vi "measure_voltage_lasers.vi"(8 "rate":dbl=100.0, 10 "number of samples":i32=100) -> (1 "data":dynamicdata(graph), 2 "Detected Voltage":string, 3 "Incident Voltage":string)   [LabVIEW 2017]
uses:
  <vilib>/Analysis/baseanly.llb/Mean (DBL).vi
  <vilib>/Analysis/NI_AALBase.lvlib
panel:
  out "Waveform Graph 2":dynamicdata(graph)
  out "Waveform Graph":dynamicdata(graph)
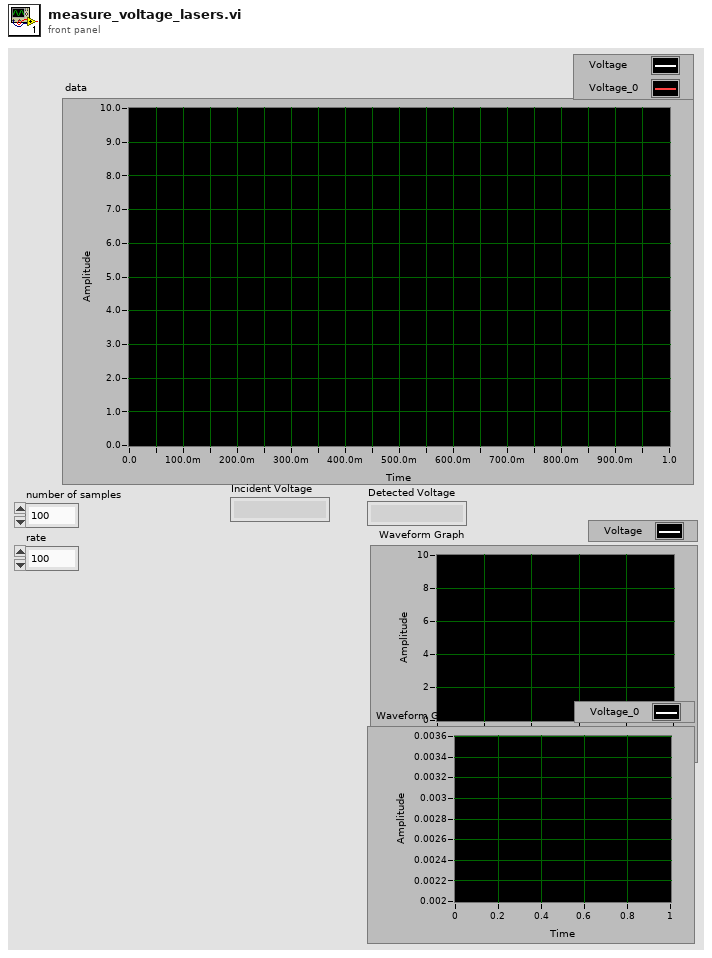
[diagram p1: front panel]
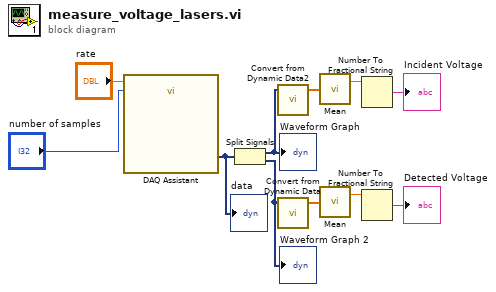
[diagram p0: block diagram]
diagram:
  n1 = call "DAQ Assistant"("rate"="rate", "number of samples"="number of samples") -> ("data"=w6:dynamicdata)  [unwired: 15 in, 2 out]
  "data" <- w6
  n2 = Split Signals(w6) -> (w5:dynamicdata, w1:dynamicdata)  [unwired: 2 in]
  "Waveform Graph" <- w5
  "Waveform Graph 2" <- w1
  n3 = call "Convert from Dynamic Data2"("Dynamic Data Type"=w5) -> ("Array"=w3:dbl[])  [unwired: 3 in]
  n4 = call "Convert from Dynamic Data"("Dynamic Data Type"=w1) -> ("Array"=w9:dbl[])  [unwired: 3 in]
  n5 = call-poly <vilib>:"Mean.vi"("X"=w3) -> ("mean"=w4:dbl)  [unwired: 1 out]
  n6 = call-poly <vilib>:"Mean.vi"("X"=w9) -> ("mean"=w8:dbl)  [unwired: 1 out]
  n7 = Number To Fractional String(number=w4) -> (F-format string=→"Incident Voltage":string)  [unwired: 3 in]
  n8 = Number To Fractional String(number=w8) -> (F-format string=→"Detected Voltage":string)  [unwired: 3 in]
